vi "Rollover2.vi"(7 "reset":bool, 8 "rollover state":T1, 11 "counter":u32[](array[numeric])) -> (0 "rollover state":T1, 3 "counter":dbl[](array[numeric]))   [LabVIEW 2017]
uses:
  <vilib>/addons/InsightCM/Utilities/Misc/rolloverState.ctl
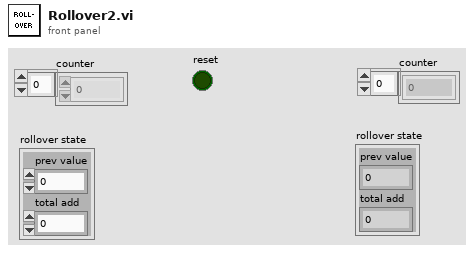
[diagram p1: front panel]
types:
  T1 = typedef "rolloverState.ctl" = cluster{"prev value":u32, "total add":dbl}
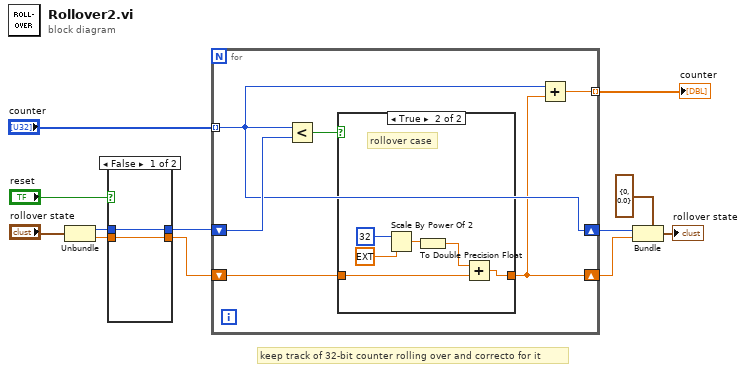
[diagram p0: block diagram]
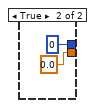
[diagram p2: hidden frame]
diagram:
  # "keep track of 32-bit counter rolling over and correcto for it"
  n1 = Unbundle("rollover state") -> ("prev value"=w4:u32, "total add"=w3:dbl)
  n2 = case shown="False" "reset" {
    tunnel: w4 -> [w14 _]
    tunnel: w3 -> [w13 _]
    tunnel: [w14 u32 0 ("tacho counts")] -> w2
    tunnel: [w13 0.0] -> w1
    frame False {
    }
    frame True {
    }
  }
  n3 = for {
    tunnel: "counter" -> [w19] mode=indexing
    shift-right: [w19] -> w10
    shift-left: w2 -> [w22]
    shift-right: [w18] -> w9
    shift-left: w1 -> [w20]
    tunnel: [w17] -> w11 mode=indexing
    n4 = Less?(x=w19, y=w22) -> (x < y?=w21:bool)
    n5 = case shown="True" w21 {
      tunnel: w20 -> [w23 w29]
      tunnel: [w23 w26] -> w18
      frame False {
      }
      frame True {
        # "rollover case"
        n6 = Scale By Power Of 2(n=i16 32, x=ext 1.0) -> (x*2^n=w25:ext)
        n7 = To Double Precision Float(number=w25) -> (double precision float=w24:dbl)
        n8 = Add(x=w24, y=w29) -> (x+y=w26:dbl)
      }
    }
    n9 = Add(x=w19, y=w18) -> (x+y=w17:dbl)
  }
  "counter" <- w11
  n10 = Bundle(cluster=T1 {"prev value"=0, "total add"=0.0}, "prev value"=w10, "total add"=w9) -> (→"rollover state":T1)
